vi "Calculate Center.vi"(8 "Type of Assembly Tray":i32, 9 "Syringe Coordinates":dbl[](array[numeric]), 10 "Relative Coordinates":dbl[][](array[numeric]), 11 "Fiducial Measurements":dbl[][](array[numeric])) -> (3 "XYZTheta Centers":dbl[][](array[numeric]))   [LabVIEW 2016, in "Assembly Tray.lvclass"]
uses:
  Assembly Tray.lvclass
panel:
  out "theta":dbl
  out "x-y":dbl
  out "x+y":dbl
  out "element":dbl
  out "appended array":dbl[](array[numeric])
  out "Relative Coordinates 2":dbl[][](array[numeric])
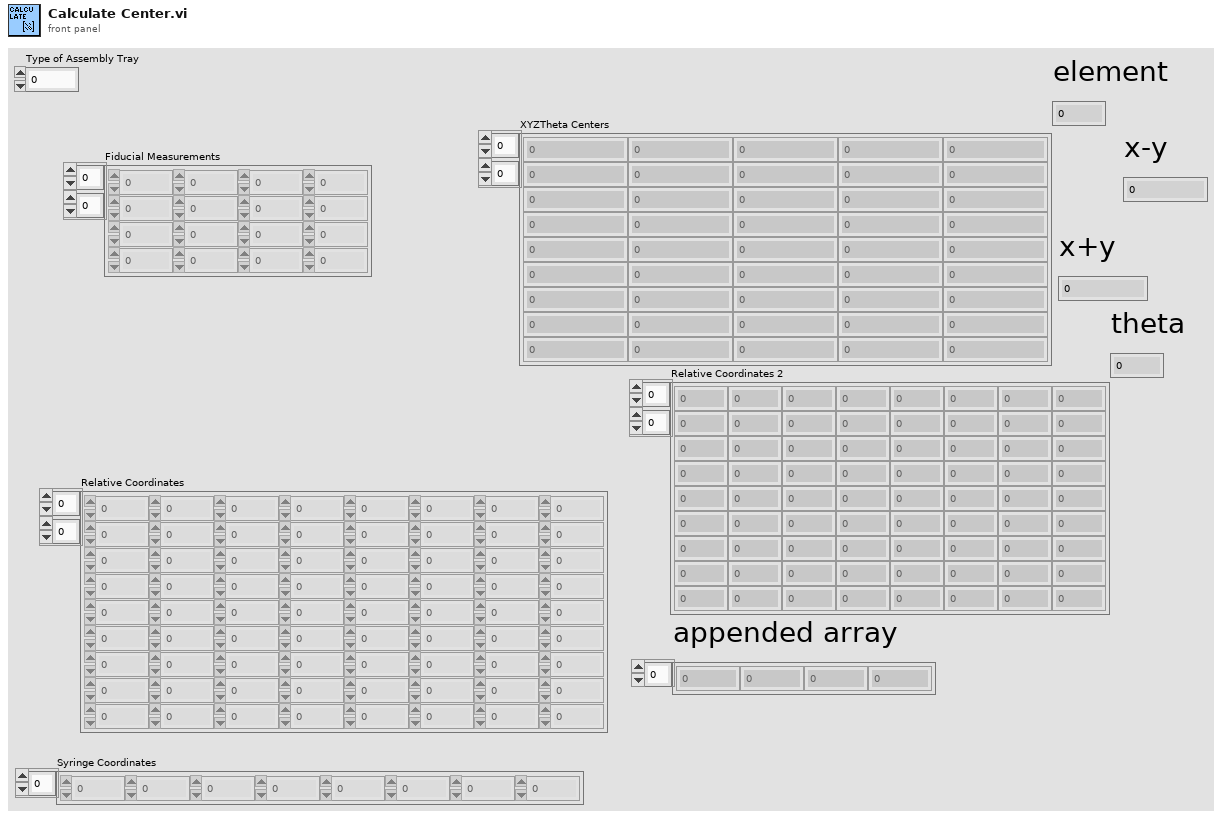
[diagram p1: front panel]
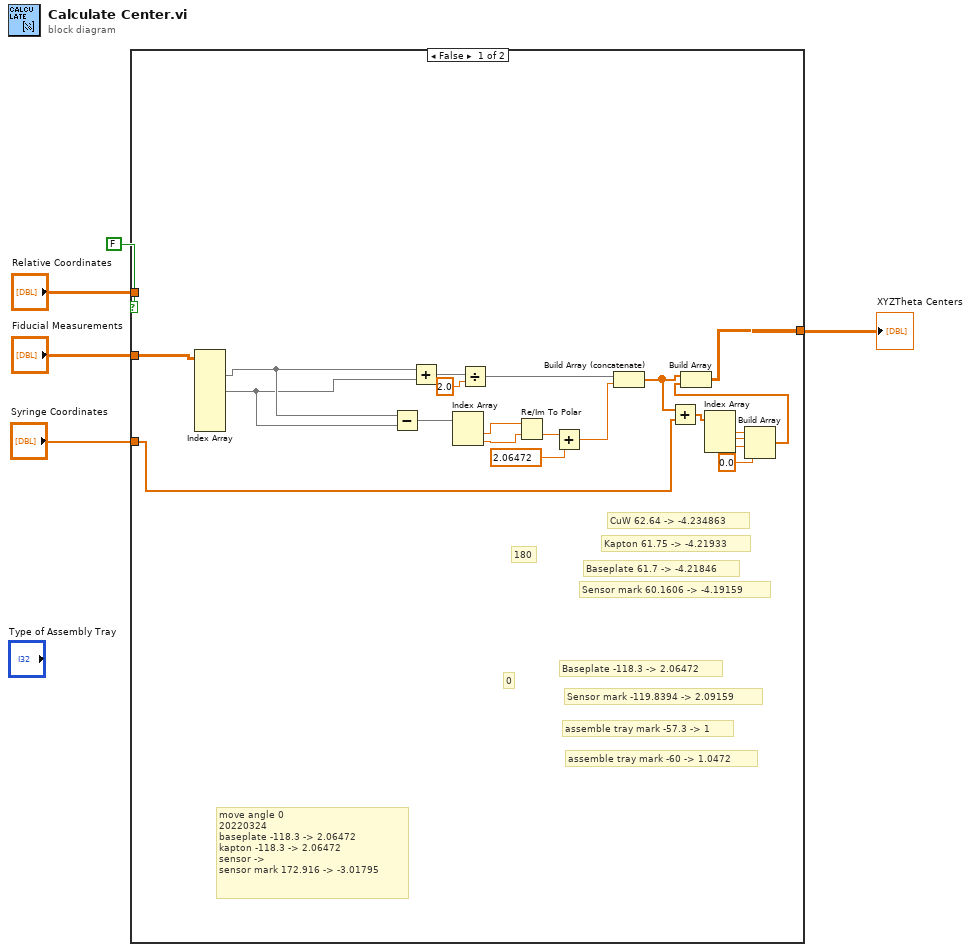
[diagram p0: block diagram]
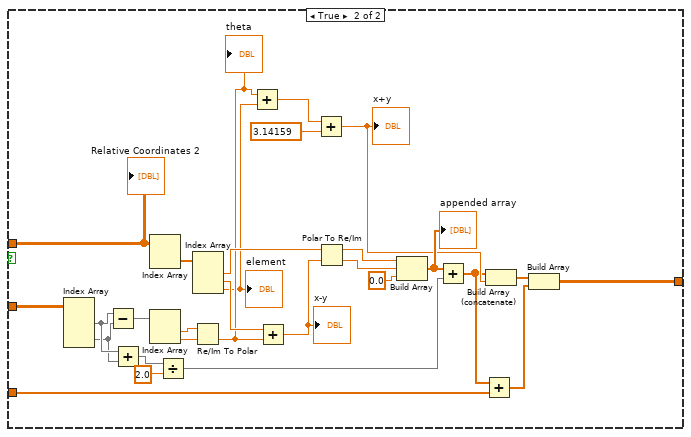
[diagram p2: hidden frame]
diagram:
  n1 = case shown="False" FALSE {
    tunnel: "Fiducial Measurements" -> [w24 w54]
    tunnel: "Relative Coordinates" -> [_ w53]
    tunnel: [w14 w38] -> w3
    tunnel: "Syringe Coordinates" -> [w12 w37]
    frame False {
      # "move angle 0\n20220324\nbaseplate -118.3 -> 2.06472\nkapton -118.3 -> 2.06472\nsensor ->\nsensor mark 172.916 -> -3.01795"
      # "0"
      # "180"
      # "assemble tray mark -60 -> 1.0472"
      # "assemble tray mark -57.3 -> 1"
      # "Sensor mark -119.8394 -> 2.09159"
      # "Baseplate -118.3 -> 2.06472"
      # "Sensor mark 60.1606 -> -4.19159"
      # "Baseplate 61.7 -> -4.21846"
      # "Kapton 61.75 -> -4.21933"
      # "CuW 62.64 -> -4.234863"
      n2 = Index Array(array=w24) -> (element #1=w23:dbl[], element #2=w22:dbl[])  [unwired: 8 in, 2 out]
      n3 = Subtract(x=w23, y=w22) -> (x-y=w21:dbl[])
      n4 = Add(x=w23, y=w22) -> (x+y=w26:dbl[])
      n5 = Index Array(array=w21) -> (element #1=w20:dbl, element #2=w19:dbl)  [unwired: 2 in]
      n6 = Divide(x=w26, y=2.0) -> (x/y=w16:dbl[])
      n7 = Re/Im To Polar(2:w19, 3:w20) -> (0:w18:dbl)  [unwired: 1 out]
      n8 = Add(x=w18, y=2.06472) -> (x+y=w15:dbl)
      n9 = Build Array (concatenate)(w16, w15) -> (w13:dbl[])
      n10 = Add(x=w13, y=w12) -> (x+y=w11:dbl[])
      n11 = Index Array(array=w11) -> (element #1=w10:dbl, element #2=w9:dbl, element #3=w8:dbl)  [unwired: 3 in]
      n12 = Build Array(w10, w9, w8, 0.0 ("element")) -> (w6:dbl[])
      n13 = Build Array(w13, w6) -> (w14:dbl[][])
    }
    frame True {
      n14 = Index Array(array=w54) -> (element #1=w31:dbl[], element #2=w30:dbl[])  [unwired: 4 in]
      n15 = Subtract(x=w31, y=w30) -> (x-y=w46:dbl[])
      n16 = Add(x=w31, y=w30) -> (x+y=w29:dbl[])
      n17 = Index Array(array=w53) -> (element=w52:dbl[])  [unwired: 2 in]
      n18 = Index Array(array=w46) -> (element #1=w42:dbl, element #2=w41:dbl)  [unwired: 2 in]
      n19 = Divide(x=w29, y=2.0) -> (x/y=w27:dbl[])
      n20 = Index Array(array=w52) -> (element #1=w49:dbl, element #2=w51:dbl, element #3=w32:dbl)  [unwired: 3 in]
      "element" <- w32
      n21 = Re/Im To Polar(2:w41, 3:w42) -> (0:w33:dbl)  [unwired: 1 out]
      "theta" <- w33
      n22 = Add(x=w33, y=w32) -> (x+y=w48:dbl)
      n23 = Add(x=w51, y=w33) -> (x+y=w50:dbl)
      "x-y" <- w50
      n24 = Add(x=w48, y=3.14159) -> (x+y=w40:dbl)
      "x+y" <- w40
      n25 = Polar To Re/Im(2:w50, 3:w49) -> (0:w44:dbl, 1:w45:dbl)
      n26 = Build Array(w45, w44, 0.0 ("element")) -> (w43:dbl[])
      "appended array" <- w43
      n27 = Add(x=w43, y=w27) -> (x+y=w36:dbl[])
      n28 = Add(x=w36, y=w37) -> (x+y=w35:dbl[])
      n29 = Build Array (concatenate)(w36, w40) -> (w39:dbl[])
      n30 = Build Array(w39, w35) -> (w38:dbl[][])
      "Relative Coordinates 2" <- w53
    }
  }
  "XYZTheta Centers" <- w3
